vi "unflattenAccelerationFromXML.vi"   [LabVIEW 2016, in "UnitsAndXML.lvlib"]
doc: "Generates time in the unit specified in <B>accelerationUnitInXML</B> from the data in <B>xmlString</B>, where the source unit is <B>accelerationUnitInXML</B>. The VI uses <B>accelerationForType</B> to select the appropriate polymorphic method."
uses:
  <userlib>/Common/UnitsAndXML/UnitsAndXML.lvlib
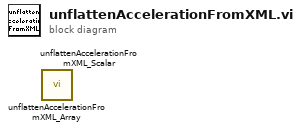
[diagram p0: block diagram]
diagram:
  n1 = call <userlib>:"unflattenAccelerationFromXML_Array.vi"() -> ()  [unwired: 10 in, 2 out]
  n2 = call <userlib>:"unflattenAccelerationFromXML_Scalar.vi"() -> ()  [unwired: 10 in, 2 out]
